vi "AppConfigTypeToXML.vi"(8 "error in (no error)":errorcluster, 11 "ModelValidation in":refnum<class "ModelValidationPlugin.lvclass">) -> (0 "error out":errorcluster, 2 "ConfigXML out":string, 3 "ModelValidation out":refnum<class "ModelValidationPlugin.lvclass">)   [LabVIEW 2017, in "AppPlugins.lvlib" / "ModelValidationPlugin.lvclass"]
uses:
  ModelValidationPlugin.lvclass
  PublicAPI/TypeDef/Config.ctl
  ModelValidationPlugin.lvclass/ModelValidationPlugin.ctl
  Accessors/Read ModelValidationConfig.vi
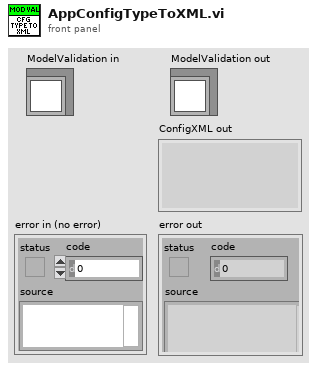
[diagram p1: front panel]
types:
  T1 = typedef "AppPlugins.lvlib/ModelValidationPlugin.lvclass/Config.ctl" = cluster{"NoiseVariance":dbl, "Iindex":i32, "OffsetTime":dbl, "InterpolationFactor":i32, "Initial condition":cluster{"H0":dbl, "xd0":dbl, "D0":dbl}}
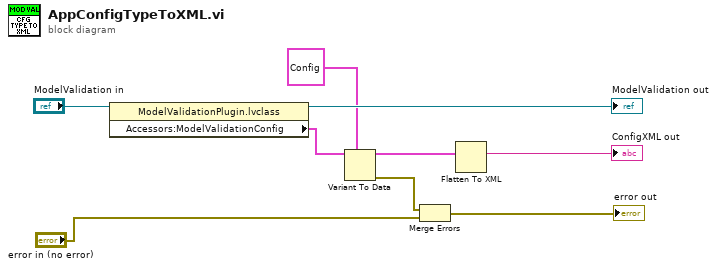
[diagram p0: block diagram]
diagram:
  n1 = property class="ModelValidationPlugin.lvclass"(reference="ModelValidation in") -> (reference out=→"ModelValidation out":refnum<class "ModelValidationPlugin.lvclass">, "Accessors:ModelValidationConfig"=w8:T1)  [unwired: 1 in, 1 out]
  n2 = Variant To Data(type=T1 {"NoiseVariance"=0.05, "Iindex"=3, "OffsetTime"=2.0, "InterpolationFactor"=3, "Initial condition"={"H0"=4.55, "xd0"=0.275, "D0"=4.2}} ("ModelValidationConfig"), Variant=w8) -> (data=w5:T1, error out=w6:errorcluster)  [unwired: 1 in]
  n3 = Merge Errors(w6, "error in (no error)") -> (→"error out":errorcluster)
  n4 = Flatten To XML(anything=w5) -> (xml string=→"ConfigXML out":string)
